vi "Add Finger Cmd.vi"(1 "ID NUMBER":u16) -> (0 "Add Cmd":string)   [LabVIEW 2020]
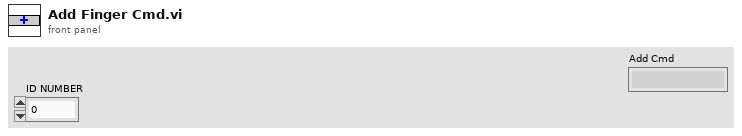
[diagram p1: front panel]
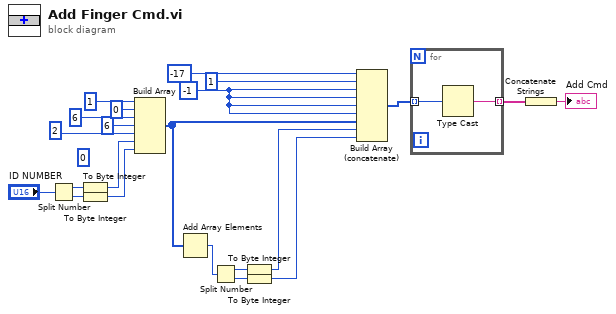
[diagram p0: block diagram]
diagram:
  (unwired) i8 0
  w12 = i8 -1
  n1 = Split Number(x="ID NUMBER") -> (hi(x)=w7:u8, lo(x)=w8:u8)
  n2 = To Byte Integer(number=w7) -> (8bit integer=w19:i8)
  n3 = To Byte Integer(number=w8) -> (8bit integer=w20:i8)
  n4 = Build Array(i8 1, i8 0, i8 6, i8 6, i8 2, w19, w20) -> (w17:i8[])
  n5 = Add Array Elements(numeric array=w17) -> (sum=w3:i8)
  n6 = Split Number(x=w3) -> (hi(x)=w5:u8, lo(x)=w4:u8)
  n7 = To Byte Integer(number=w5) -> (8bit integer=w2:i8)
  n8 = To Byte Integer(number=w4) -> (8bit integer=w1:i8)
  n9 = Build Array (concatenate)(i8 -17, i8 1, w12, w12, w12, w12, w17, w2, w1) -> (w22:i8[])
  n10 = for {
    tunnel: [w24] -> w21 mode=indexing
    tunnel: w22 -> [w23] mode=indexing
    n11 = Type Cast(x=w23) -> (*(type *) &x=w24:string)  [unwired: 1 in]
  }
  n12 = Concatenate Strings(w21) -> (→"Add Cmd":string)
